vi "Execution Report.vi"(8 "error in (no error)":errorcluster, 10 "Execution":refnum<class "Execution.lvclass">, 11 "Engine in":refnum<class "Engine.lvclass">) -> (0 "error out":errorcluster, 2 "Report":refnum<class "Report.lvclass">, 3 "Engine out":refnum<class "Engine.lvclass">)   [LabVIEW 2020, in "TSnax.lvlib" / "Engine.lvclass"]
uses:
  Engine.lvclass
  Engine.lvclass/Engine.ctl
  Execution/Execution.lvclass
  Report/Report.lvclass
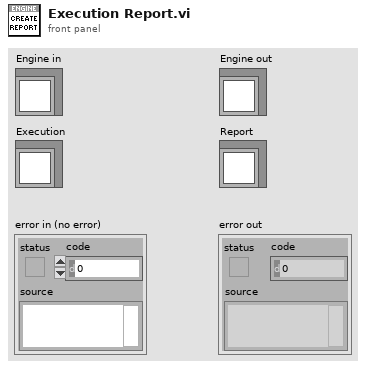
[diagram p1: front panel]
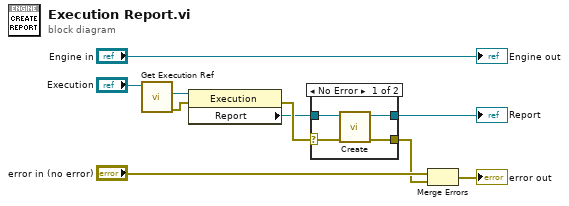
[diagram p0: block diagram]
diagram:
  n1 = call "Get Execution Ref.vi"("Execution in"="Execution") -> ("error out"=w4:errorcluster, "Execution Ref"=w6:refnum<k7>)  [unwired: 8 in, 1 out]
  n2 = property class="Execution"(reference=w6, error in=w4) -> (error out=w10:errorcluster, "Report"=w5:refnum<k7>)  [unwired: 1 out]
  n3 = case shown="No Error" w10 {
    selector: w10 -> [w14 w15]
    tunnel: w5 -> [w13 _]
    tunnel: [w12 w15] -> w2
    tunnel: [w11 _] -> w1
    frame No Error {
      n4 = call "Create.vi"("error in (no error)"=w14, "Report Ref"=w13) -> ("error out"=w12:errorcluster, "Report out"=w11:refnum<class "Report.lvclass">)  [unwired: 8 in]
    }
    frame Error {
    }
  }
  "Report" <- w1
  n5 = Merge Errors("error in (no error)", w2) -> (→"error out":errorcluster)
  "Engine out" <- "Engine in"
